vi "BallTrackingSub.vi"(7 "Rectangle":T2 {"Rotation" min=-90.0 max=90.0 step=1.0 format="%.2f"; "Left" scale=0.0..1024.0; "Right" scale=0.0..1024.0}, 8 "error in (no error)":errorcluster, 9 "Match Options":T3 {"Range Settings"."Match Constraints" items=["Rotation Angle (degrees)", "Scale Factor (%)", "Occlusion (%)"]}, 10 "Circle Descriptor":cluster{"Min Radius":dbl, "Max Radius":dbl}={"Min Radius"=3.0, "Max Radius"=500.0}, 11 "Refnum in":T1) -> (0 "error out":errorcluster, 3 "Position":cluster{"X":sgl, "Y":sgl})   [LabVIEW 2021]
uses:
  <vilib>/vision/Shape Detection.llb/ShapeDetectionMatchOptions.ctl
  <vilib>/vision/Pattern Matching.llb/IMAQ Match Range Setting.ctl
  <vilib>/userDefined/High Color/IMAQdx.ctl
  <vilib>/vision/driver/IMAQdx.llb/IMAQdx Acquisition Mode.ctl
  <vilib>/vision/driver/IMAQdx.llb/IMAQdx Buffer Number Mode.ctl
  <vilib>/vision/Management.llb/Cast Image 2 Method.ctl
  <vilib>/vision/driver/NI_Vision_Acquisition_Software.lvlib
  <vilib>/vision/NI_Vision_Development_Module.lvlib
panel:
  # "Range"
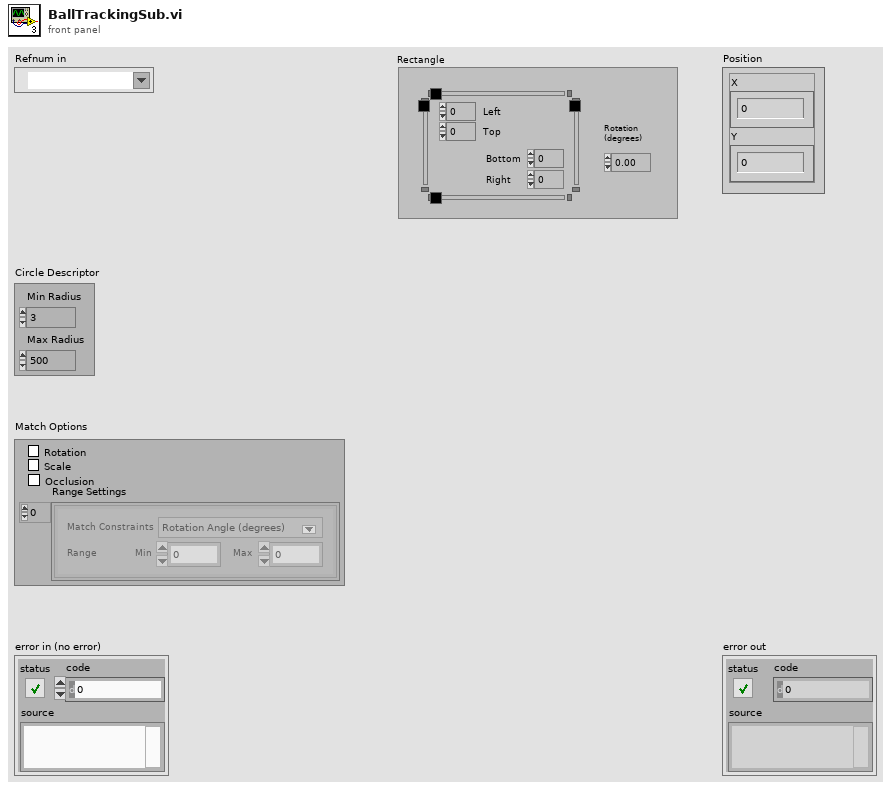
[diagram p1: front panel]
types:
  T1 = typedef "IMAQdx.ctl" = refnum<k21>
  T2 = typedef "IMAQ Rectangle" = cluster{"Left":i32, "Top":i32, "Right":i32, "Bottom":i32, "Rotation":dbl}
  T3 = typedef "ShapeDetectionMatchOptions.ctl" = cluster{"Rotation":bool, "Scale":bool, "Occlusion":bool, "Range Settings":T4[]}
  T4 = typedef "IMAQ Match Range Setting.ctl" = cluster{"Match Constraints":u32, "Min":dbl, "Max":dbl}
  T5 = typedef "Image Type" = u32
  T6 = typedef "NI_Vision_Acquisition_Software.lvlib/IMAQdx Acquisition Mode.ctl" = enum32{"One Shot", "Continuous"}
  T7 = typedef "IMAQ Image.ctl" = refnum<image>
  T8 = typedef "NI_Vision_Acquisition_Software.lvlib/IMAQdx Buffer Number Mode.ctl" = enum32{"Next", "Last", "Buffer Number", "Every", "Last New"}
  T9 = typedef "Cast Image 2 Method.ctl" = u32
  T10 = typedef "ROI Descriptor" = cluster{"Global Rectangle":i32[], "Contours":cluster{"ID":enum32{"External", "Internal"}, "Type":u32, "Coordinates":i32[]}[]}
  T11 = cluster{"Position":cluster{"X":sgl, "Y":sgl}, "Radius":dbl, "Score":dbl}[]
  T12 = cluster{"Position":cluster{"X":sgl, "Y":sgl}, "Radius":dbl, "Score":dbl}
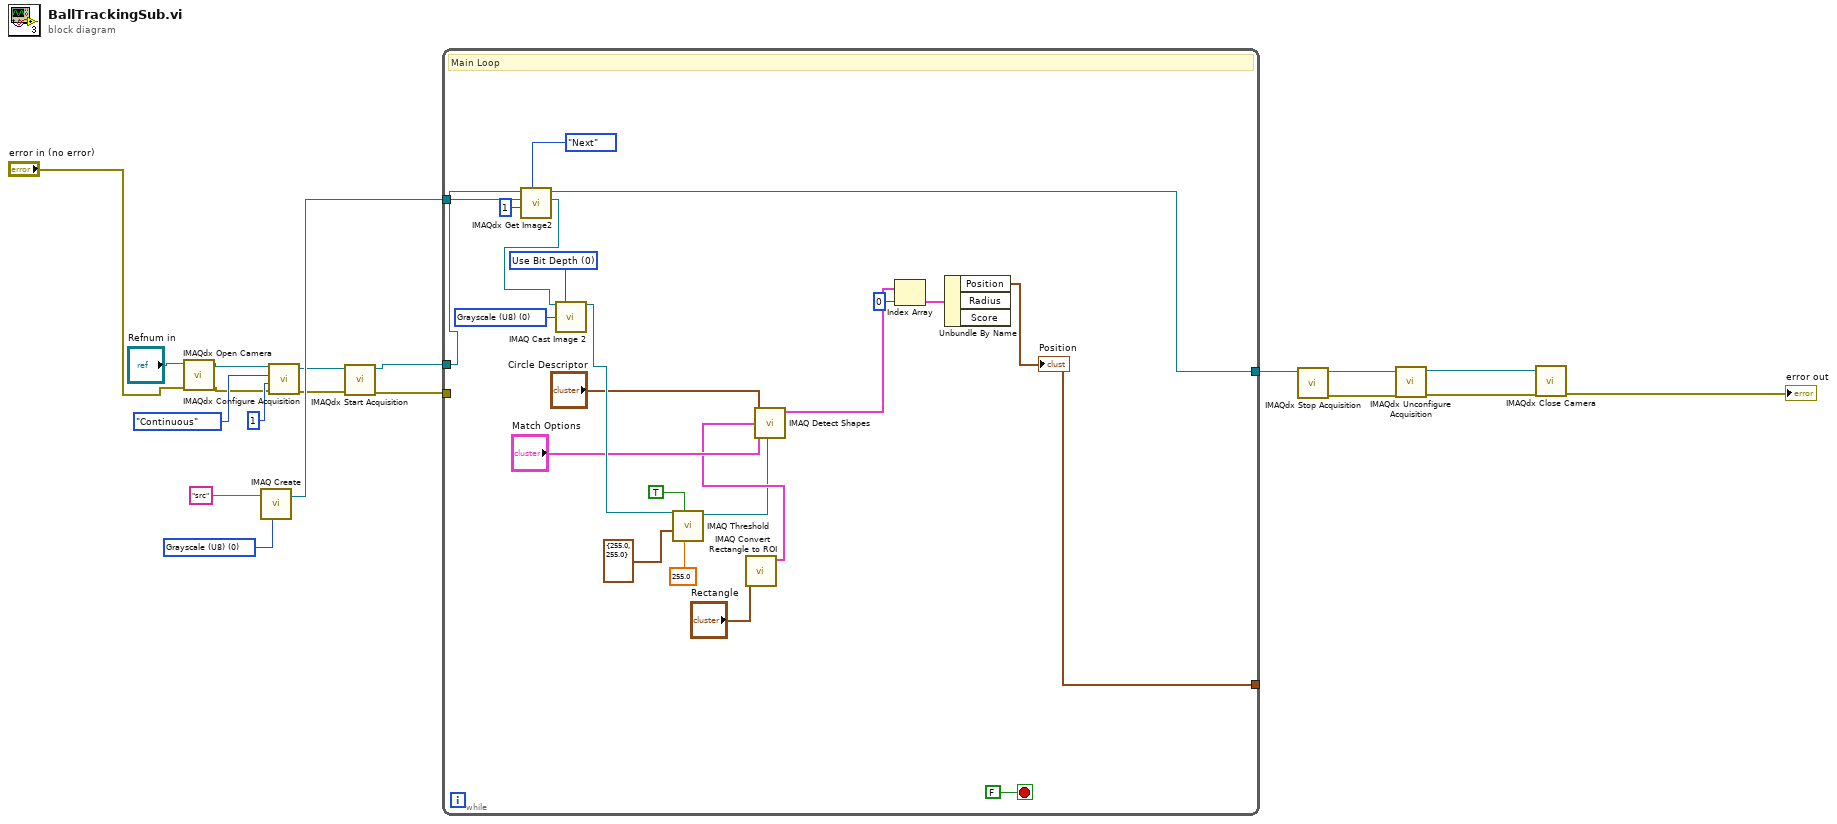
[diagram p0: block diagram]
diagram:
  w18 = T5 0 items=["Grayscale (U8)", "Grayscale (I16)", "Grayscale (SGL)", "Complex (CSG)", "RGB (U32)", "HSL (U32)", "RGB (U64)", "Grayscale (U16)"] ("Image Type")
  n1 = call <vilib>:"IMAQdx Open Camera.vi"("error in"="error in (no error)", "Session In"="Refnum in") -> ("error out"=w10:errorcluster, "Session Out"=w9:T1)  [unwired: 8 in]
  n2 = call "IMAQ Create"("Image Name"="src", "Image Type"=w18) -> ("New Image"=w19:T7)  [unwired: 3 in, 1 out]
  n3 = call <vilib>:"IMAQdx Configure Acquisition.vi"("error in"=w10, "Number of Buffers"=u32 1, "Continuous?"=IMAQdx_Acquisition_Mode."Continuous", "Session In"=w9) -> ("error out"=w1:errorcluster, "Session Out"=w2:T1)  [unwired: 6 in]
  n4 = call <vilib>:"IMAQdx Start Acquisition.vi"("error in"=w1, "Session In"=w2) -> ("error out"=w3:errorcluster, "Session Out"=w4:T1)  [unwired: 8 in]
  n5 = while {
    tunnel: w4 -> [w27]
    tunnel: w3 -> [_]
    tunnel: [w29] -> w16
    tunnel: w19 -> [w26]
    tunnel: [w20] -> _
    stop <- FALSE stop-if-true
    w38 = T9 0 items=["Use Bit Depth", "Shift", "Use Lookup Table"] ("Method")
    w39 = T5 0 items=["Grayscale (U8)", "Grayscale (I16)", "Grayscale (SGL)", "Complex (CSG)", "RGB (U32)", "HSL (U32)", "RGB (U64)", "Grayscale (U16)"] ("Image Type")
    # "Main Loop"
    n6 = call <vilib>:"IMAQdx Get Image2.vi"("Buffer Number Mode (Next)"=IMAQdx_Buffer_Number_Mode."Next", "Buffer Number In"=u32 1, "Image In"=w26, "Session In"=w27) -> ("Image Out"=w21:T7, "Session Out"=w29:T1)  [unwired: 4 in, 2 out]
    n7 = call "IMAQ Cast Image 2"("Image Src"=w21, "Method"=w38, "Image Type"=w39) -> ("Image Dst Out"=w37:T7)  [unwired: 11 in, 1 out]
    n8 = call "IMAQ Threshold"("Replace Value"=sgl 255.0, "Keep/Replace Value (Replace)"=TRUE, "Range"=cluster{"Upper value":sgl, "Lower value":sgl} {"Upper value"=255.0, "Lower value"=255.0}, "Image Src"=w37) -> ("Image Dst Out"=w30:T7)  [unwired: 6 in, 1 out]
    n9 = call "IMAQ Convert Rectangle to ROI"("Rectangle"="Rectangle") -> ("ROI Descriptor"=w31:T10)  [unwired: 8 in, 1 out]
    n10 = call-poly "IMAQ Detect Shapes"("ROI Descriptor"=w31, "Match Options"="Match Options", "Circle Descriptor"="Circle Descriptor", "Image"=w30) -> ("Circles"=w24:T11)  [unwired: 5 in, 2 out]
    n11 = Index Array(array=w24, index=0) -> (element=w22:T12)
    n12 = Unbundle By Name(w22) -> ("Position"=w20:cluster{"X":sgl, "Y":sgl})  [unwired: 2 out]
    "Position" <- w20
  }
  n13 = call <vilib>:"IMAQdx Stop Acquisition.vi"("Session In"=w16) -> ("error out"=w7:errorcluster, "Session Out"=w8:T1)  [unwired: 9 in]
  n14 = call <vilib>:"IMAQdx Unconfigure Acquisition.vi"("error in"=w7, "Session In"=w8) -> ("error out"=w5:errorcluster, "Session Out"=w6:T1)  [unwired: 8 in]
  n15 = call <vilib>:"IMAQdx Close Camera.vi"("error in"=w5, "Session In"=w6) -> ("error out"=→"error out":errorcluster)  [unwired: 9 in]
